vi "Enable Multiple Boolean Controls.vi"(8 "error in (no error)":errorcluster, 10 "Enabled":bool=TRUE, 11 "References":refnum<vi>[](array[refnum])) -> (0 "error out":errorcluster)   [LabVIEW 2014]
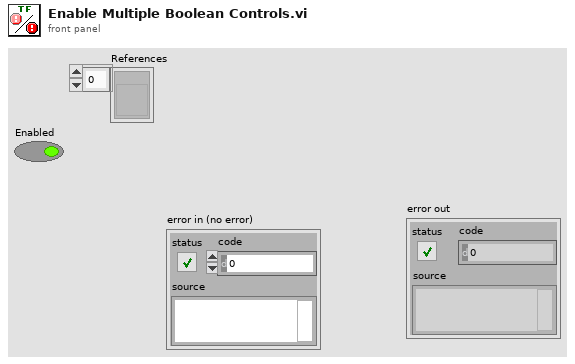
[diagram p1: front panel]
types:
  T1 = enum8{"Enabled", "Disabled", "Disabled and Grayed Out"}
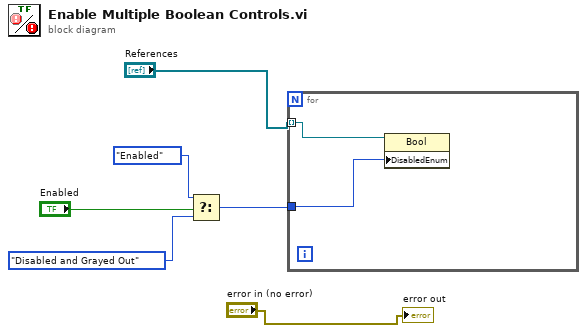
[diagram p0: block diagram]
diagram:
  n1 = Select(t=T1."Enabled" ("Disabled"), s="Enabled", f=T1."Disabled and Grayed Out" ("Disabled")) -> (s? t:f=w2:T1)
  n2 = for {
    tunnel: "References" -> [w8] mode=indexing
    tunnel: w2 -> [w7]
    n3 = property class="Bool"(reference=w8, "DisabledEnum"=w7) -> ()  [unwired: 1 in, 2 out]
  }
  "error out" <- "error in (no error)"
